vi "MecanumRobot.vi"() -> ()   [LabVIEW 2019]
uses:
  <vilib>/MakerHub/Xbox-One-Controller/Public/Open First Controller.vi
  <vilib>/vision/driver/NI_Vision_Acquisition_Software.lvlib
  <vilib>/MakerHub/Xbox-One-Controller/Private/Type Defs/Indicators/DPad Enum.ctl
  <vilib>/MakerHub/Xbox-One-Controller/Private/Type Defs/Indicators/All Axis Data.ctl
panel:
  out "SALIDA 4":string
  in  "Tab Control":enum32{"JOYSTICK", "COMUNICACION", "CAMARA"}(tab)
  out "A":bool
  out "AB":bool
  out "B":bool
  out "stay":bool
  out "Reverse":bool
  out "Forward":bool
  out "Left":bool
  out "Right":bool
  out "RL":bool
  out "FR":bool
  out "RR":bool
  out "FL":bool
  out "All Axis":T1
  out "Boolean":bool
  in  "Boton Prueba":bool
  in  "BOTON A":bool
  out "SALIDA":string
  out "SALIDA 2":string
  in  "address":string="192.168.0.16"
  out "SALIDA 3":string
  in  "stop":bool
  in  "DETENER EL PROGRAMA":bool
  out "Buffer Number":u32
  out "Frame Rate":dbl(knob) scale=0.0..100.0
  in  "Stop":bool
  in  "Camera Name":refnum<k21> caption="IMAQdx Session"
  out "Image":T3(plugin-control)
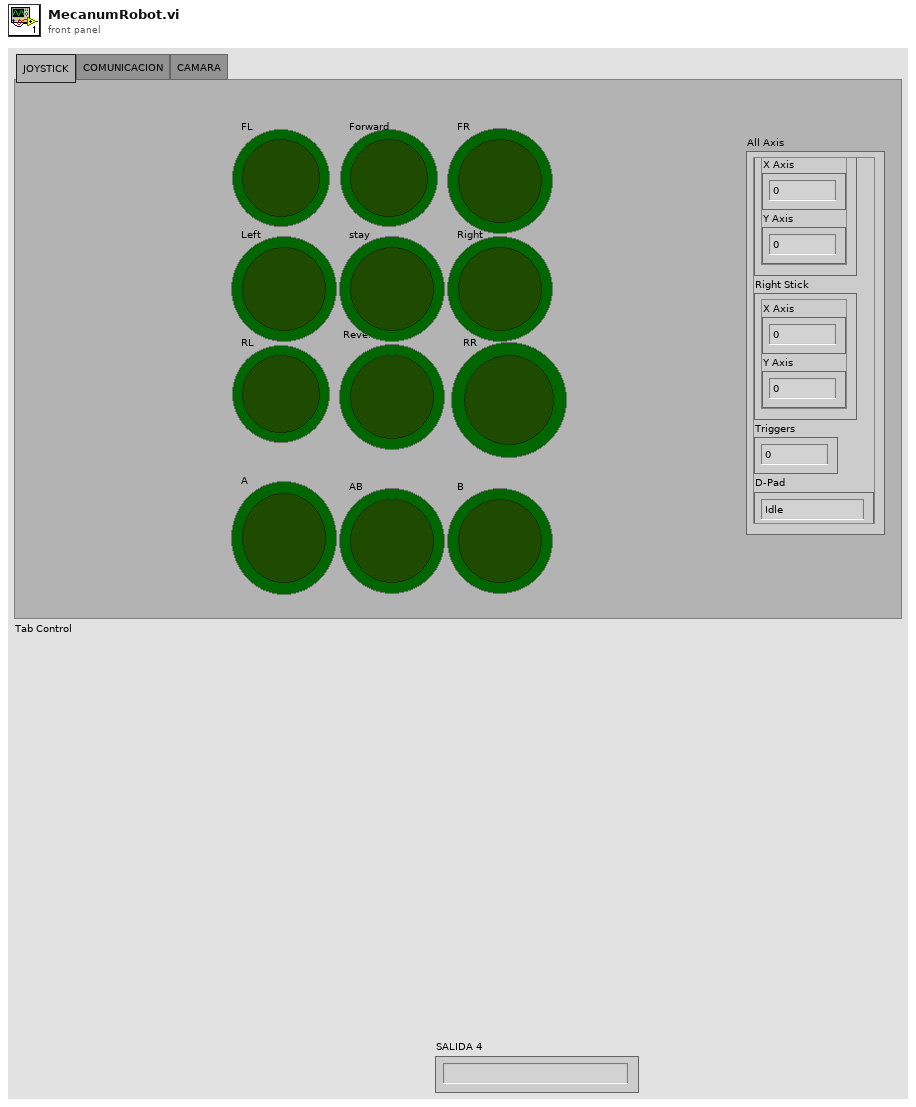
[diagram p1: front panel]
types:
  T1 = typedef "LMH-Xbox-One-Controller.lvlib/All Axis Data.ctl" = cluster{"Left Stick":cluster{"X Axis":i32, "Y Axis":i32}, "Right Stick":cluster{"X Axis":i32, "Y Axis":i32}, "Triggers":i32, "D-Pad":T2}
  T2 = typedef "LMH-Xbox-One-Controller.lvlib/DPad Enum.ctl" = enum16{"Idle", "Up", "Up / Right", "Right", "Down / Right", "Down", "Down / Left", "Left", "Up / Left"}
  T3 = typedef "IMAQ Image.ctl" = refnum<image>
  T4 = typedef "LMH-Xbox-One-Controller.lvlib/Xbox One Controller Ref.ctl" = cluster{"Controller Ref":refnum<k1>, "Event Refnum":refnum<event-registration>, "Worker Ref":refnum<vi>}
  T5 = typedef "IMAQdx.ctl" = refnum<k21>
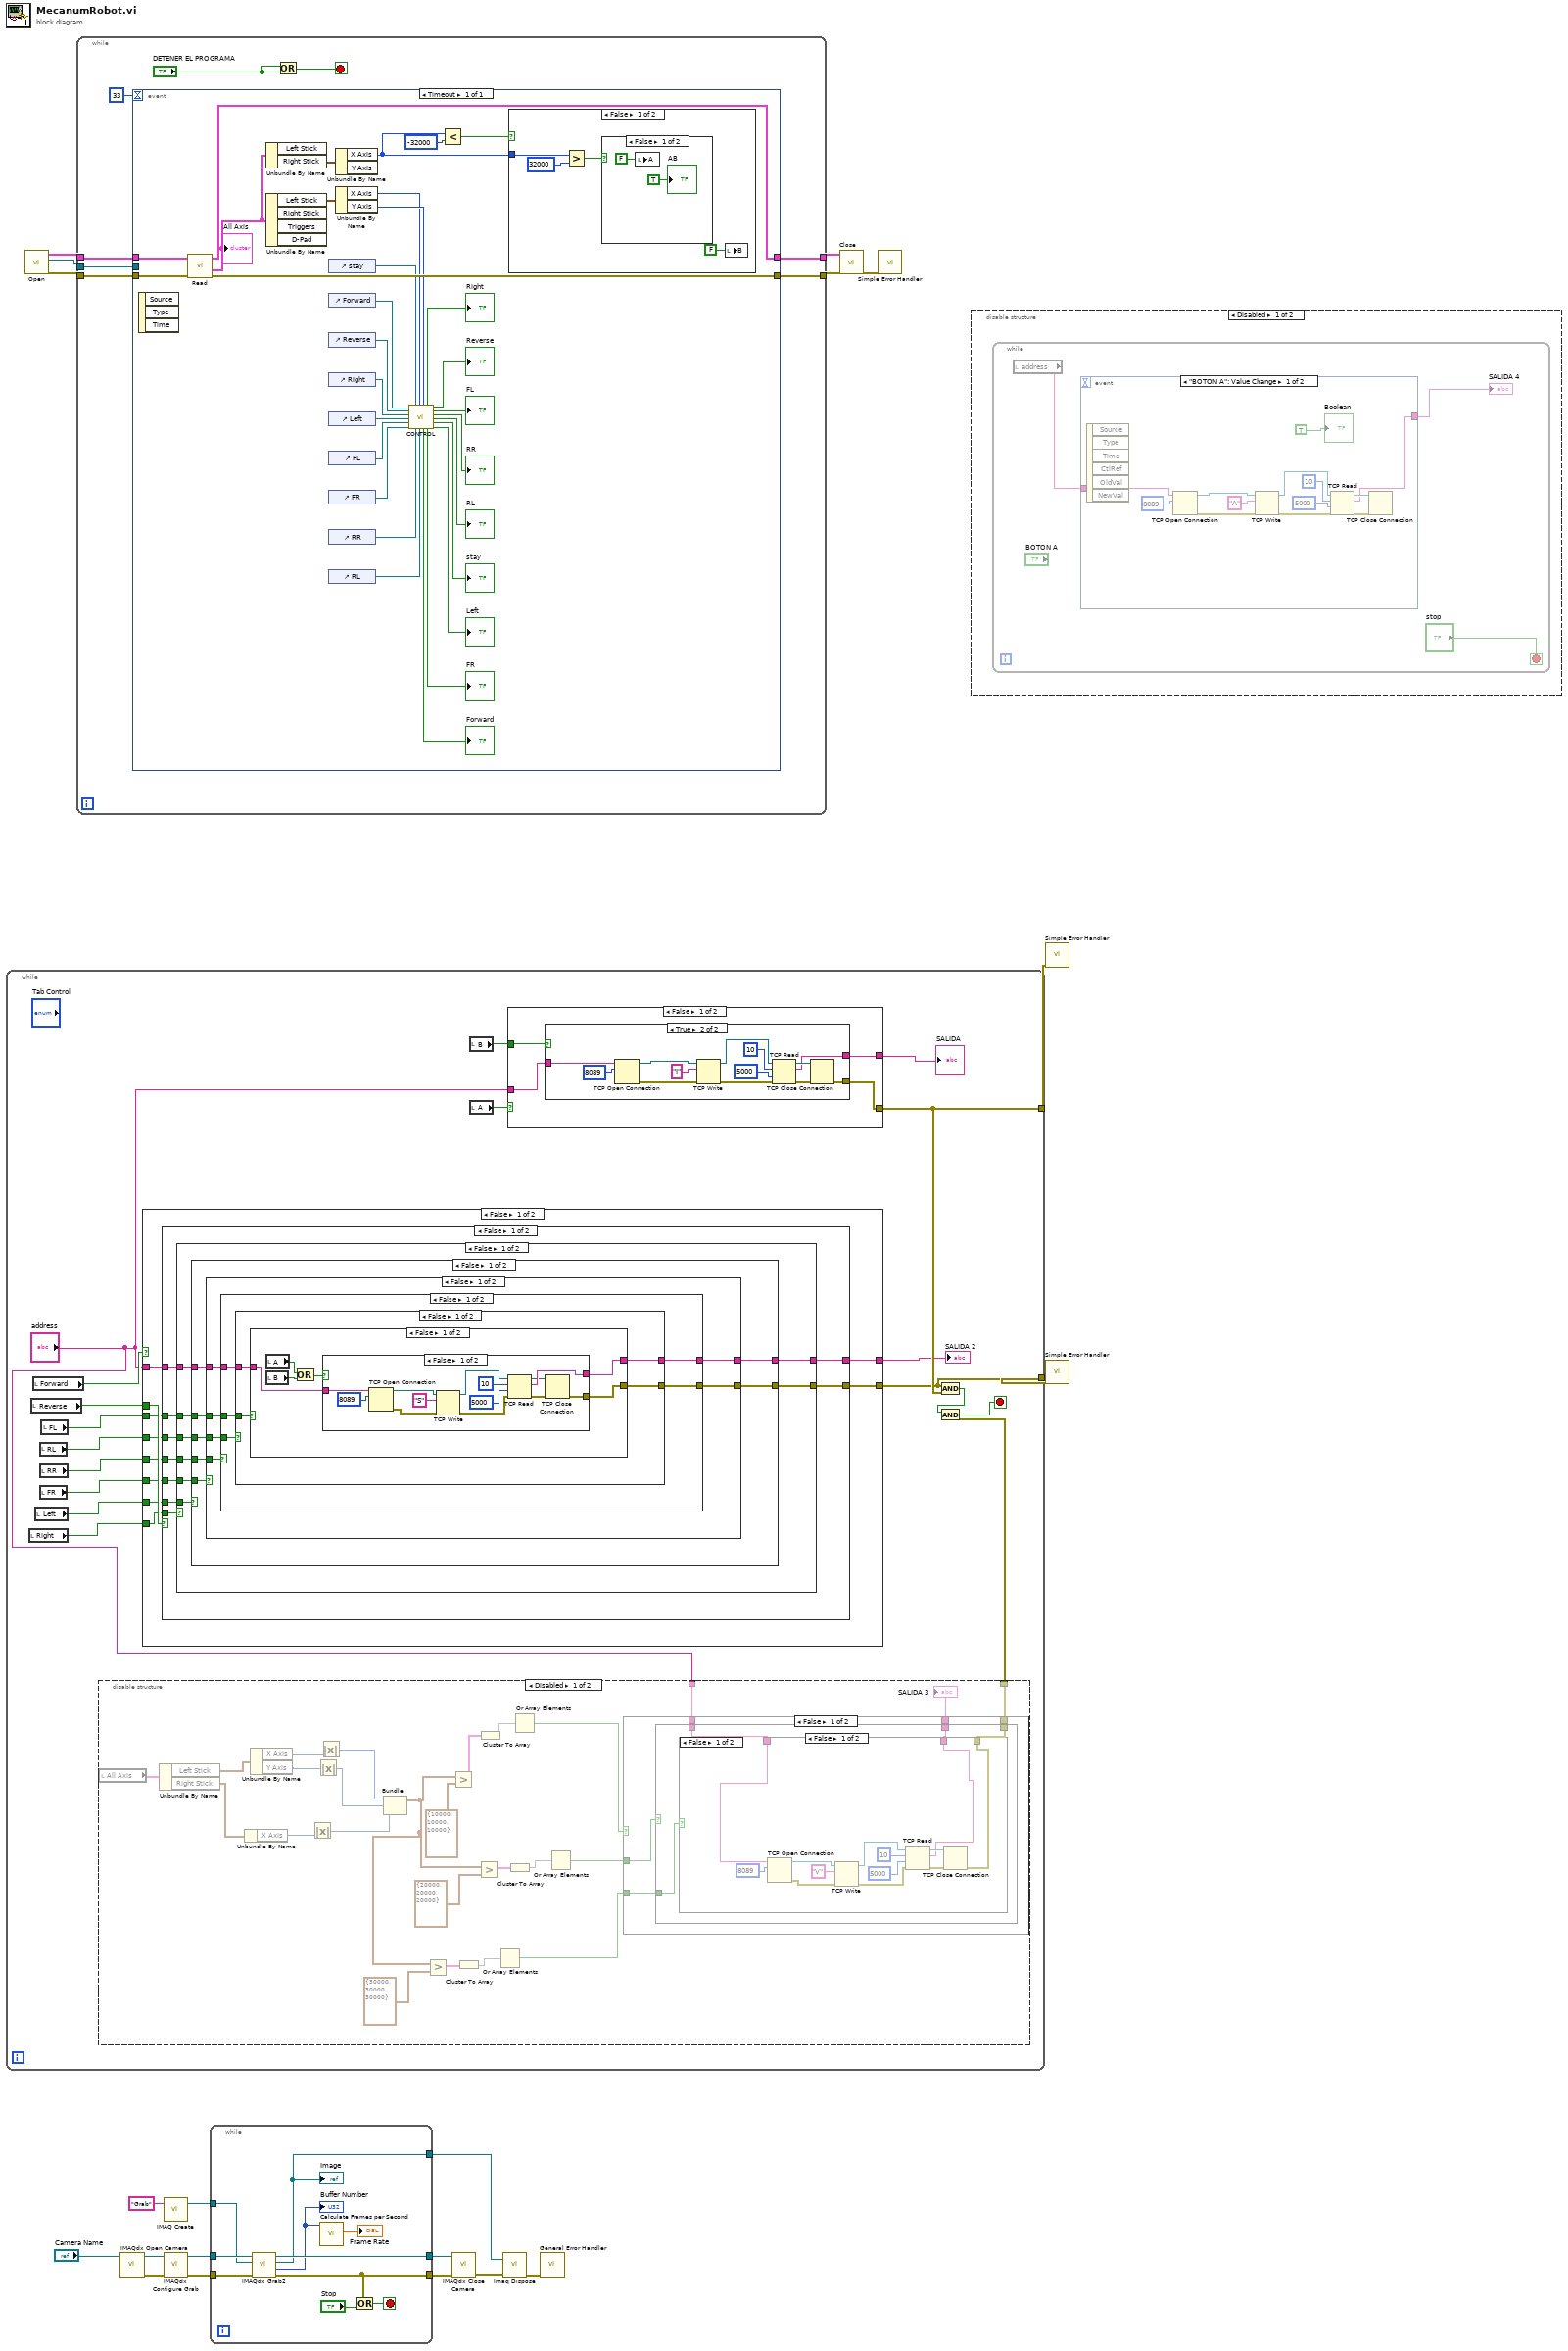
[diagram p0: block diagram]
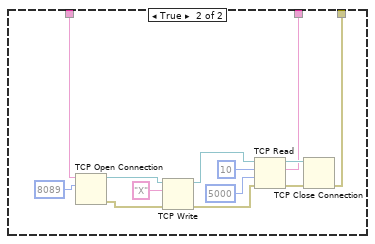
[diagram p2: hidden frame]
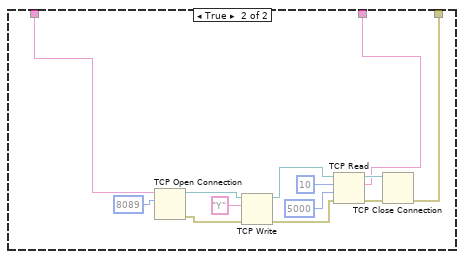
[diagram p3: hidden frame]
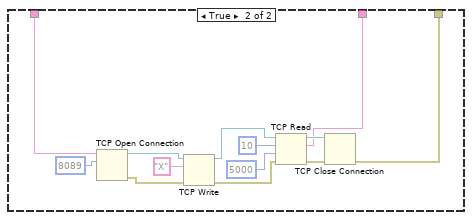
[diagram p4: hidden frame]
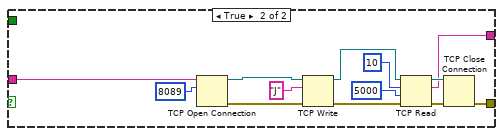
[diagram p7: hidden frame]
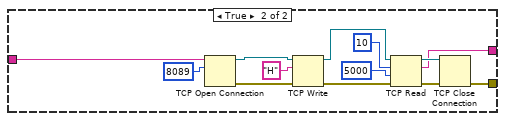
[diagram p9: hidden frame]
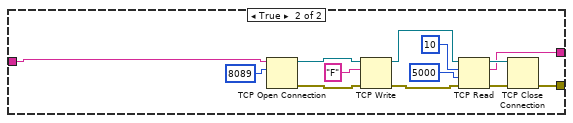
[diagram p10: hidden frame]
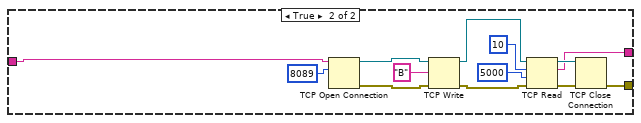
[diagram p11: hidden frame]
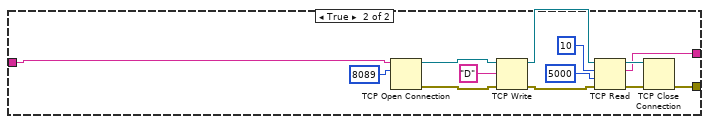
[diagram p12: hidden frame]
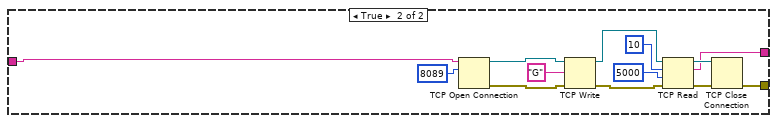
[diagram p13: hidden frame]
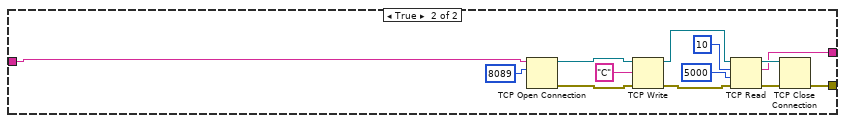
[diagram p14: hidden frame]
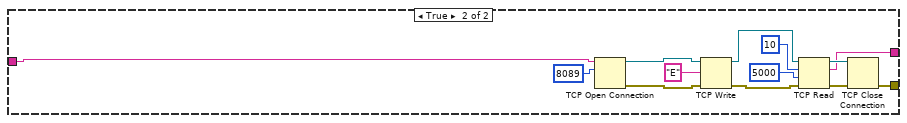
[diagram p15: hidden frame]
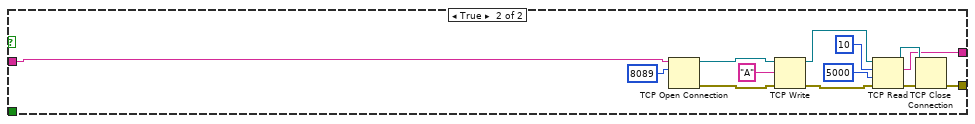
[diagram p16: hidden frame]
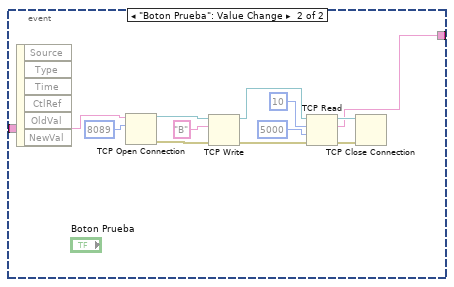
[diagram p17: hidden frame]
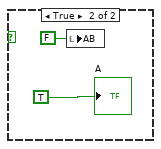
[diagram p19: hidden frame]
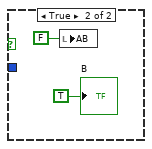
[diagram p20: hidden frame]
diagram:
  n1 = while {
    tunnel: [w28] -> w13
    tunnel: [w29] -> w14
    stop <- w21 stop-if-true
    n2 = local read "Right"() -> (w36:bool)
    n3 = local read "Reverse"() -> (w37:bool)
    n4 = local read "Forward"() -> (w38:bool)
    n5 = local read "Left"() -> (w35:bool)
    n6 = local read "RL"() -> (w32:bool)
    n7 = local read "RR"() -> (w33:bool)
    n8 = local read "FR"() -> (w34:bool)
    n9 = local read "FL"() -> (w31:bool)
    n10 = disable-structure shown="Disabled" {
      disable-tunnel: "address" -> [w63 _]
      disable-tunnel: [w62 _] -> w22
      frame Disabled {
        n11 = local read "All Axis"() -> (w61:T1)
        n12 = Unbundle By Name(w61) -> ("Left Stick"=w60:cluster{"X Axis":i32, "Y Axis":i32}, "Right Stick"=w59:cluster{"X Axis":i32, "Y Axis":i32})
        n13 = Unbundle By Name(w59) -> ("X Axis"=w53:i32)
        n14 = Unbundle By Name(w60) -> ("X Axis"=w58:i32, "Y Axis"=w57:i32)
        n15 = Absolute Value(x=w53) -> (abs(x)=w54:i32)
        n16 = Absolute Value(x=w57) -> (abs(x)=w55:i32)
        n17 = Absolute Value(x=w58) -> (abs(x)=w56:i32)
        n18 = Bundle(w56, w55, w54) -> (w43:cluster{i32, i32, i32})  [unwired: 1 in]
        n19 = Greater?(x=w43, y=cluster{i32, i32, i32} {30000, 30000, 30000}) -> (0:w45:cluster{bool, bool, bool})
        n20 = Greater?(x=w43, y=cluster{i32, i32, i32} {10000, 10000, 10000}) -> (0:w51:cluster{bool, bool, bool})
        n21 = Cluster To Array(cluster=w45) -> (array=w44:bool[])
        n22 = Greater?(x=w43, y=cluster{i32, i32, i32} {20000, 20000, 20000}) -> (0:w48:cluster{bool, bool, bool})
        n23 = Cluster To Array(cluster=w51) -> (array=w50:bool[])
        n24 = Or Array Elements(Boolean array=w44) -> (logical OR=w39:bool)
        n25 = Cluster To Array(cluster=w48) -> (array=w47:bool[])
        n26 = Or Array Elements(Boolean array=w50) -> (logical OR=w42:bool)
        n27 = Or Array Elements(Boolean array=w47) -> (logical OR=w40:bool)
        n28 = case shown="False" w42 {
          tunnel: w63 -> [w66 w114]
          tunnel: [w68 w113] -> w62
          tunnel: [w67 w112] -> w41
          tunnel: w40 -> [w65 _]
          tunnel: w39 -> [w64 _]
          frame False {
            n29 = case shown="False" w65 {
              tunnel: [w70 w101] -> w68
              tunnel: [w71 w100] -> w67
              tunnel: w66 -> [w69 w99]
              tunnel: w64 -> [w72 _]
              frame False {
                n30 = case shown="False" w72 {
                  tunnel: [w74 w88] -> w71
                  tunnel: [w75 w87] -> w70
                  tunnel: w69 -> [w73 w86]
                  frame False {
                    n31 = TCP Open Connection(address=w73, remote port or service name=u16 8089) -> (connection ID=w80:refnum<k5>, error out=w79:errorcluster)  [unwired: 3 in]
                    n32 = TCP Write(connection ID=w80, data in="V", error in (no error)=w79) -> (connection ID out=w83:refnum<k5>, error out=w82:errorcluster)  [unwired: 1 in, 1 out]
                    n33 = TCP Read(connection ID=w83, bytes to read=10, error in (no error)=w82, 9:5000 ("timeout ms (25000)")) -> (connection ID out=w78:refnum<k5>, data out=w74:string, error out=w77:errorcluster)  [unwired: 1 in]
                    n34 = TCP Close Connection(connection ID=w78, error in (no error)=w77) -> (error out=w75:errorcluster)  [unwired: 1 in, 1 out]
                  }
                  frame True {
                    n35 = TCP Open Connection(address=w86, remote port or service name=u16 8089) -> (connection ID=w95:refnum<k5>, error out=w96:errorcluster)  [unwired: 3 in]
                    n36 = TCP Write(connection ID=w95, data in="X", error in (no error)=w96) -> (connection ID out=w93:refnum<k5>, error out=w94:errorcluster)  [unwired: 1 in, 1 out]
                    n37 = TCP Read(connection ID=w93, bytes to read=10, error in (no error)=w94, 9:5000 ("timeout ms (25000)")) -> (connection ID out=w97:refnum<k5>, data out=w88:string, error out=w98:errorcluster)  [unwired: 1 in]
                    n38 = TCP Close Connection(connection ID=w97, error in (no error)=w98) -> (error out=w87:errorcluster)  [unwired: 1 in, 1 out]
                  }
                }
              }
              frame True {
                n39 = TCP Open Connection(address=w99, remote port or service name=u16 8089) -> (connection ID=w106:refnum<k5>, error out=w105:errorcluster)  [unwired: 3 in]
                n40 = TCP Write(connection ID=w106, data in="Y", error in (no error)=w105) -> (connection ID out=w109:refnum<k5>, error out=w108:errorcluster)  [unwired: 1 in, 1 out]
                n41 = TCP Read(connection ID=w109, bytes to read=10, error in (no error)=w108, 9:5000 ("timeout ms (25000)")) -> (connection ID out=w104:refnum<k5>, data out=w100:string, error out=w103:errorcluster)  [unwired: 1 in]
                n42 = TCP Close Connection(connection ID=w104, error in (no error)=w103) -> (error out=w101:errorcluster)  [unwired: 1 in, 1 out]
              }
            }
          }
          frame True {
            n43 = TCP Open Connection(address=w114, remote port or service name=u16 8089) -> (connection ID=w119:refnum<k5>, error out=w118:errorcluster)  [unwired: 3 in]
            n44 = TCP Write(connection ID=w119, data in="X", error in (no error)=w118) -> (connection ID out=w122:refnum<k5>, error out=w121:errorcluster)  [unwired: 1 in, 1 out]
            n45 = TCP Read(connection ID=w122, bytes to read=10, error in (no error)=w121, 9:5000 ("timeout ms (25000)")) -> (connection ID out=w117:refnum<k5>, data out=w112:string, error out=w116:errorcluster)  [unwired: 1 in]
            n46 = TCP Close Connection(connection ID=w117, error in (no error)=w116) -> (error out=w113:errorcluster)  [unwired: 1 in, 1 out]
          }
        }
        "SALIDA 3" <- w41
      }
      frame Enabled {
      }
    }
    n47 = case shown="False" w38 {
      tunnel: [w164 w316] -> w28
      tunnel: w37 -> [w163 _]
      tunnel: "address" -> [w162 w315]
      tunnel: w36 -> [w161 _]
      tunnel: w35 -> [w160 _]
      tunnel: w34 -> [w159 _]
      tunnel: w33 -> [w158 _]
      tunnel: w32 -> [w157 _]
      tunnel: w31 -> [w156 _]
      tunnel: [w155 w314] -> w26
      frame False {
        n48 = case shown="False" w163 {
          tunnel: [w172 w303] -> w164
          tunnel: w162 -> [w173 w302]
          tunnel: w161 -> [w171 _]
          tunnel: w160 -> [w170 _]
          tunnel: w159 -> [w169 _]
          tunnel: w158 -> [w168 _]
          tunnel: w157 -> [w167 _]
          tunnel: w156 -> [w166 _]
          tunnel: [w165 w301] -> w155
          frame False {
            n49 = case shown="False" w171 {
              tunnel: w173 -> [w181 w290]
              tunnel: [w180 w289] -> w172
              tunnel: w170 -> [w179 _]
              tunnel: w169 -> [w178 _]
              tunnel: w168 -> [w177 _]
              tunnel: w167 -> [w176 _]
              tunnel: w166 -> [w175 _]
              tunnel: [w174 w288] -> w165
              frame False {
                n50 = case shown="False" w179 {
                  tunnel: w181 -> [w188 w278]
                  tunnel: [w186 w276] -> w180
                  tunnel: w178 -> [w187 _]
                  tunnel: w177 -> [w185 _]
                  tunnel: w176 -> [w184 _]
                  tunnel: w175 -> [w183 _]
                  tunnel: [w182 w275] -> w174
                  frame False {
                    n51 = case shown="False" w187 {
                      tunnel: w188 -> [w193 w264]
                      tunnel: [w194 w263] -> w186
                      tunnel: w185 -> [w192 _]
                      tunnel: w184 -> [w191 _]
                      tunnel: w183 -> [w190 _]
                      tunnel: [w189 w262] -> w182
                      frame False {
                        n52 = case shown="False" w192 {
                          tunnel: [w199 w251] -> w194
                          tunnel: w193 -> [w198 w250]
                          tunnel: w191 -> [w197 _]
                          tunnel: w190 -> [w196 _]
                          tunnel: [w195 w249] -> w189
                          frame False {
                            n53 = case shown="False" w197 {
                              tunnel: [w203 w238] -> w199
                              tunnel: w198 -> [w201 w237]
                              tunnel: w196 -> [w202 _]
                              tunnel: [w200 w236] -> w195
                              frame False {
                                n54 = case shown="False" w202 {
                                tunnel: [w208 w225] -> w203
                                tunnel: w201 -> [w209 w224]
                                tunnel: [w207 w223] -> w200
                                frame False {
                                n55 = local read "A"() -> (w205:bool)
                                n56 = local read "B"() -> (w204:bool)
                                n57 = Or(x=w205, y=w204) -> (x .or. y?=w206:bool)
                                n58 = case shown="False" w206 {
                                tunnel: w209 -> [w222 _]
                                tunnel: [w221 _] -> w208
                                tunnel: [w220 _] -> w207
                                frame False {
                                n59 = TCP Open Connection(address=w222, remote port or service name=u16 8089) -> (connection ID=w214:refnum<k5>, error out=w213:errorcluster)  [unwired: 3 in]
                                n60 = TCP Write(connection ID=w214, data in="S", error in (no error)=w213) -> (connection ID out=w217:refnum<k5>, error out=w216:errorcluster)  [unwired: 1 in, 1 out]
                                n61 = TCP Read(connection ID=w217, bytes to read=10, error in (no error)=w216, 9:5000 ("timeout ms (25000)")) -> (connection ID out=w212:refnum<k5>, data out=w220:string, error out=w211:errorcluster)  [unwired: 1 in]
                                n62 = TCP Close Connection(connection ID=w212, error in (no error)=w211) -> (error out=w221:errorcluster)  [unwired: 1 in, 1 out]
                                }
                                frame True {
                                }
                                }
                                }
                                frame True {
                                n63 = TCP Open Connection(address=w224, remote port or service name=u16 8089) -> (connection ID=w230:refnum<k5>, error out=w229:errorcluster)  [unwired: 3 in]
                                n64 = TCP Write(connection ID=w230, data in="H", error in (no error)=w229) -> (connection ID out=w233:refnum<k5>, error out=w232:errorcluster)  [unwired: 1 in, 1 out]
                                n65 = TCP Read(connection ID=w233, bytes to read=10, error in (no error)=w232, 9:5000 ("timeout ms (25000)")) -> (connection ID out=w228:refnum<k5>, data out=w223:string, error out=w227:errorcluster)  [unwired: 1 in]
                                n66 = TCP Close Connection(connection ID=w228, error in (no error)=w227) -> (error out=w225:errorcluster)  [unwired: 1 in, 1 out]
                                }
                                }
                              }
                              frame True {
                                n67 = TCP Open Connection(address=w237, remote port or service name=u16 8089) -> (connection ID=w243:refnum<k5>, error out=w242:errorcluster)  [unwired: 3 in]
                                n68 = TCP Write(connection ID=w243, data in="F", error in (no error)=w242) -> (connection ID out=w246:refnum<k5>, error out=w245:errorcluster)  [unwired: 1 in, 1 out]
                                n69 = TCP Read(connection ID=w246, bytes to read=10, error in (no error)=w245, 9:5000 ("timeout ms (25000)")) -> (connection ID out=w241:refnum<k5>, data out=w236:string, error out=w240:errorcluster)  [unwired: 1 in]
                                n70 = TCP Close Connection(connection ID=w241, error in (no error)=w240) -> (error out=w238:errorcluster)  [unwired: 1 in, 1 out]
                              }
                            }
                          }
                          frame True {
                            n71 = TCP Open Connection(address=w250, remote port or service name=u16 8089) -> (connection ID=w258:refnum<k5>, error out=w259:errorcluster)  [unwired: 3 in]
                            n72 = TCP Write(connection ID=w258, data in="B", error in (no error)=w259) -> (connection ID out=w256:refnum<k5>, error out=w257:errorcluster)  [unwired: 1 in, 1 out]
                            n73 = TCP Read(connection ID=w256, bytes to read=10, error in (no error)=w257, 9:5000 ("timeout ms (25000)")) -> (connection ID out=w260:refnum<k5>, data out=w249:string, error out=w261:errorcluster)  [unwired: 1 in]
                            n74 = TCP Close Connection(connection ID=w260, error in (no error)=w261) -> (error out=w251:errorcluster)  [unwired: 1 in, 1 out]
                          }
                        }
                      }
                      frame True {
                        n75 = TCP Open Connection(address=w264, remote port or service name=u16 8089) -> (connection ID=w271:refnum<k5>, error out=w272:errorcluster)  [unwired: 3 in]
                        n76 = TCP Write(connection ID=w271, data in="D", error in (no error)=w272) -> (connection ID out=w269:refnum<k5>, error out=w270:errorcluster)  [unwired: 1 in, 1 out]
                        n77 = TCP Read(connection ID=w269, bytes to read=10, error in (no error)=w270, 9:5000 ("timeout ms (25000)")) -> (connection ID out=w273:refnum<k5>, data out=w262:string, error out=w274:errorcluster)  [unwired: 1 in]
                        n78 = TCP Close Connection(connection ID=w273, error in (no error)=w274) -> (error out=w263:errorcluster)  [unwired: 1 in, 1 out]
                      }
                    }
                  }
                  frame True {
                    n79 = TCP Open Connection(address=w278, remote port or service name=u16 8089) -> (connection ID=w282:refnum<k5>, error out=w281:errorcluster)  [unwired: 3 in]
                    n80 = TCP Write(connection ID=w282, data in="G", error in (no error)=w281) -> (connection ID out=w285:refnum<k5>, error out=w284:errorcluster)  [unwired: 1 in, 1 out]
                    n81 = TCP Read(connection ID=w285, bytes to read=10, error in (no error)=w284, 9:5000 ("timeout ms (25000)")) -> (connection ID out=w280:refnum<k5>, data out=w275:string, error out=w279:errorcluster)  [unwired: 1 in]
                    n82 = TCP Close Connection(connection ID=w280, error in (no error)=w279) -> (error out=w276:errorcluster)  [unwired: 1 in, 1 out]
                  }
                }
              }
              frame True {
                n83 = TCP Open Connection(address=w290, remote port or service name=u16 8089) -> (connection ID=w294:refnum<k5>, error out=w293:errorcluster)  [unwired: 3 in]
                n84 = TCP Write(connection ID=w294, data in="C", error in (no error)=w293) -> (connection ID out=w298:refnum<k5>, error out=w297:errorcluster)  [unwired: 1 in, 1 out]
                n85 = TCP Read(connection ID=w298, bytes to read=10, error in (no error)=w297, 9:5000 ("timeout ms (25000)")) -> (connection ID out=w292:refnum<k5>, data out=w288:string, error out=w291:errorcluster)  [unwired: 1 in]
                n86 = TCP Close Connection(connection ID=w292, error in (no error)=w291) -> (error out=w289:errorcluster)  [unwired: 1 in, 1 out]
              }
            }
          }
          frame True {
            n87 = TCP Open Connection(address=w302, remote port or service name=u16 8089) -> (connection ID=w307:refnum<k5>, error out=w306:errorcluster)  [unwired: 3 in]
            n88 = TCP Write(connection ID=w307, data in="E", error in (no error)=w306) -> (connection ID out=w311:refnum<k5>, error out=w310:errorcluster)  [unwired: 1 in, 1 out]
            n89 = TCP Read(connection ID=w311, bytes to read=10, error in (no error)=w310, 9:5000 ("timeout ms (25000)")) -> (connection ID out=w305:refnum<k5>, data out=w301:string, error out=w304:errorcluster)  [unwired: 1 in]
            n90 = TCP Close Connection(connection ID=w305, error in (no error)=w304) -> (error out=w303:errorcluster)  [unwired: 1 in, 1 out]
          }
        }
      }
      frame True {
        n91 = TCP Open Connection(address=w315, remote port or service name=u16 8089) -> (connection ID=w320:refnum<k5>, error out=w319:errorcluster)  [unwired: 3 in]
        n92 = TCP Write(connection ID=w320, data in="A", error in (no error)=w319) -> (connection ID out=w324:refnum<k5>, error out=w323:errorcluster)  [unwired: 1 in, 1 out]
        n93 = TCP Read(connection ID=w324, bytes to read=10, error in (no error)=w323, 9:5000 ("timeout ms (25000)")) -> (connection ID out=w318:refnum<k5>, data out=w314:string, error out=w317:errorcluster)  [unwired: 1 in]
        n94 = TCP Close Connection(connection ID=w318, error in (no error)=w317) -> (error out=w316:errorcluster)  [unwired: 1 in, 1 out]
      }
    }
    "SALIDA 2" <- w26
    n95 = local read "B"() -> (w27:bool)
    n96 = local read "A"() -> (w30:bool)
    n97 = case shown="False" w30 {
      tunnel: [w126 w144] -> w29
      tunnel: "address" -> [w127 w143]
      tunnel: w27 -> [w128 _]
      tunnel: [w125 w142] -> w25
      frame False {
        n98 = case shown="True" w128 {
          tunnel: w127 -> [_ w131]
          tunnel: [_ w130] -> w126
          tunnel: [_ w129] -> w125
          frame False {
          }
          frame True {
            n99 = TCP Open Connection(address=w131, remote port or service name=u16 8089) -> (connection ID=w139:refnum<k5>, error out=w138:errorcluster)  [unwired: 3 in]
            n100 = TCP Write(connection ID=w139, data in="I", error in (no error)=w138) -> (connection ID out=w141:refnum<k5>, error out=w140:errorcluster)  [unwired: 1 in, 1 out]
            n101 = TCP Read(connection ID=w141, bytes to read=10, error in (no error)=w140, 9:5000 ("timeout ms (25000)")) -> (connection ID out=w137:refnum<k5>, data out=w129:string, error out=w136:errorcluster)  [unwired: 1 in]
            n102 = TCP Close Connection(connection ID=w137, error in (no error)=w136) -> (error out=w130:errorcluster)  [unwired: 1 in, 1 out]
          }
        }
      }
      frame True {
        n103 = TCP Open Connection(address=w143, remote port or service name=u16 8089) -> (connection ID=w151:refnum<k5>, error out=w152:errorcluster)  [unwired: 3 in]
        n104 = TCP Write(connection ID=w151, data in="J", error in (no error)=w152) -> (connection ID out=w149:refnum<k5>, error out=w150:errorcluster)  [unwired: 1 in, 1 out]
        n105 = TCP Read(connection ID=w149, bytes to read=10, error in (no error)=w150, 9:5000 ("timeout ms (25000)")) -> (connection ID out=w153:refnum<k5>, data out=w142:string, error out=w154:errorcluster)  [unwired: 1 in]
        n106 = TCP Close Connection(connection ID=w153, error in (no error)=w154) -> (error out=w144:errorcluster)  [unwired: 1 in, 1 out]
      }
    }
    "SALIDA" <- w25
    n107 = And(x=w28, y=w29) -> (x .and. y?=w23:bool)
    n108 = And(x=w23, y=w22) -> (x .and. y?=w21:bool)
  }
  n109 = call-poly <vilib>:"Open.vi"() -> ("Error Out"=w18:errorcluster, "Event Refnum"=w19:refnum<event-registration>, "Xbox One Controller"=w20:T4)  [unwired: 9 in]
  n110 = while {
    tunnel: w20 -> [w334]
    tunnel: w19 -> [w333]
    tunnel: w18 -> [w332]
    tunnel: [w331] -> w17
    tunnel: [w330] -> w16
    stop <- w328 stop-if-true
    n111 = event shown="[0] Timeout" {
      selector: _ -> [_]
      dyn-events: _ -> [_]
      timeout: 33 -> [_]
      tunnel: w334 -> [w363]
      tunnel: w333 -> [_]
      tunnel: w332 -> [w364]
      tunnel: [w340] -> w331
      tunnel: [w362] -> w330
      event Timeout {
        n112 = event-data() -> ()  [unwired: 1 in, 3 out]
        n113 = call <vilib>:"Read.vi"("Error In"=w364, "Xbox One Controller Ref"=w363) -> ("Error Out"=w362:errorcluster, "All Axis"=w339:T1, "Xbox One Controller Ref"=w340:T4)  [unwired: 6 in, 1 out]
        "All Axis" <- w339
        n114 = Unbundle By Name(w339) -> ("Right Stick"=w338:cluster{"X Axis":i32, "Y Axis":i32})  [unwired: 1 out]
        n115 = Unbundle By Name(w339) -> ("Left Stick"=w361:cluster{"X Axis":i32, "Y Axis":i32})  [unwired: 3 out]
        n116 = control-ref of="stay"() -> (w351:refnum<vi>)
        n117 = control-ref of="Forward"() -> (w350:refnum<vi>)
        n118 = control-ref of="Reverse"() -> (w358:refnum<vi>)
        n119 = control-ref of="Right"() -> (w357:refnum<vi>)
        n120 = control-ref of="Left"() -> (w356:refnum<vi>)
        n121 = control-ref of="FL"() -> (w355:refnum<vi>)
        n122 = control-ref of="FR"() -> (w354:refnum<vi>)
        n123 = control-ref of="RR"() -> (w353:refnum<vi>)
        n124 = control-ref of="RL"() -> (w352:refnum<vi>)
        n125 = Unbundle By Name(w338) -> ("X Axis"=w335:i32)  [unwired: 1 out]
        n126 = Unbundle By Name(w361) -> ("X Axis"=w359:i32, "Y Axis"=w360:i32)
        n127 = call "CONTROL.vi"("Boolean in"=w350, "reference"=w358, "reference 2"=w357, "reference 3"=w356, "reference 4"=w355, "reference 5"=w354, "reference 8"=w351, "reference 6"=w353, "X Axis"=w359, "reference 7"=w352, "Y Axis"=w360) -> ("Foward"=→"Forward":bool, "Right"=→"Right":bool, "FR"=→"FR":bool, "Reverse"=→"Reverse":bool, "FL"=→"FL":bool, "RR"=→"RR":bool, "RL"=→"RL":bool, "stay"=→"stay":bool, "Left"=→"Left":bool)
        n128 = Less?(x=w335, y=-32000) -> (x < y?=w336:bool)
        n129 = case shown="False" w336 {
          tunnel: w335 -> [w368 _]
          frame False {
            n130 = Greater?(x=w368, y=32000) -> (0:w366:bool)
            n131 = case shown="False" w366 {
              frame False {
                n132 = local write "A"(FALSE ("A")) -> ()
                "AB" <- TRUE ("AB")
              }
              frame True {
                n133 = local write "AB"(FALSE ("AB")) -> ()
                "A" <- TRUE ("A")
              }
            }
            n134 = local write "B"(FALSE ("A")) -> ()
          }
          frame True {
            n135 = local write "AB"(FALSE ("AB")) -> ()
            "B" <- TRUE ("B")
          }
        }
      }
    }
    n136 = Or(x="DETENER EL PROGRAMA", y="DETENER EL PROGRAMA") -> (x .or. y?=w328:bool)
  }
  n137 = call <vilib>:"IMAQdx Open Camera.vi"("Session In"="Camera Name") -> ("error out"=w7:errorcluster, "Session Out"=w6:T5)  [unwired: 2 in, 7 out]
  n138 = call "IMAQ Create"("Image Name"="Grab") -> ("New Image"=w12:T3)  [unwired: 3 in, 2 out]
  n139 = call <vilib>:"IMAQdx Configure Grab.vi"("error in"=w7, "Session In"=w6) -> ("error out"=w10:errorcluster, "Session Out"=w11:T5)  [unwired: 1 in, 7 out]
  n140 = while {
    tunnel: [w379] -> w9
    tunnel: w10 -> [w381]
    tunnel: w11 -> [w382]
    tunnel: [w376] -> w8
    tunnel: w12 -> [w380]
    tunnel: [w375] -> w4
    stop <- w384 stop-if-true
    n141 = call <vilib>:"IMAQdx Grab2.vi"("error in"=w381, "Image In"=w380, "Session In"=w382) -> ("error out"=w376:errorcluster, "Buffer Number Out"=w377:u32, "Image Out"=w375:T3, "Session Out"=w379:T5)  [unwired: 5 in]
    "Image" <- w375
    "Buffer Number" <- w377
    n142 = call <vilib>:"Calculate Frames per Second.vi"("Buffer Number"=w377) -> ("Processed Frames/s"=→"Frame Rate":dbl)  [unwired: 8 in, 2 out]
    n143 = Or(x=w376, y="Stop") -> (x .or. y?=w384:bool)
  }
  n144 = call <vilib>:"IMAQdx Close Camera.vi"("error in"=w8, "Session In"=w9) -> ("error out"=w3:errorcluster)  [unwired: 9 out]
  n145 = call "Imaq Dispose"("Image"=w4, "error in (no error)"=w3) -> ("error out"=w2:errorcluster)  [unwired: 4 in]
  n146 = call <vilib>:"General Error Handler.vi"("error in (no error)"=w2) -> ()  [unwired: 2 in, 13 out]
  n147 = call <vilib>:"Close.vi"("Error In"=w16, "Xbox One Controller Ref"=w17) -> ("Error Out"=w15:errorcluster)  [unwired: 9 in]
  n148 = call <vilib>:"Simple Error Handler.vi"("error in (no error)"=w15) -> ()  [unwired: 4 in, 5 out]
  n149 = disable-structure shown="Disabled" {
    frame Disabled {
      n150 = while {
        stop <- "stop" stop-if-true
        n151 = local read "address"() -> (w386:string)
        n152 = event shown="[0] \"BOTON A\": Value Change" {
          selector: _ -> [_ _]
          dyn-events: _ -> [_ _]
          timeout: _ -> [_ _]
          tunnel: [w390 w402] -> w387
          tunnel: w386 -> [w389 w401]
          event "BOTON A": Value Change {
            n153 = event-data() -> ()  [unwired: 1 in, 6 out]
            n154 = TCP Open Connection(address=w389, remote port or service name=u16 8089) -> (connection ID=w398:refnum<k5>, error out=w397:errorcluster)  [unwired: 3 in]
            n155 = TCP Write(connection ID=w398, data in="A", error in (no error)=w397) -> (connection ID out=w400:refnum<k5>, error out=w399:errorcluster)  [unwired: 1 in, 1 out]
            n156 = TCP Read(connection ID=w400, bytes to read=10, error in (no error)=w399, 9:5000 ("timeout ms (25000)")) -> (connection ID out=w396:refnum<k5>, data out=w390:string, error out=w395:errorcluster)  [unwired: 1 in]
            n157 = TCP Close Connection(connection ID=w396, error in (no error)=w395) -> ()  [unwired: 1 in, 2 out]
            "Boolean" <- TRUE ("Boolean")
          }
          event "Boton Prueba": Value Change {
            n158 = event-data() -> ()  [unwired: 1 in, 6 out]
            n159 = TCP Open Connection(address=w401, remote port or service name=u16 8089) -> (connection ID=w410:refnum<k5>, error out=w409:errorcluster)  [unwired: 3 in]
            n160 = TCP Write(connection ID=w410, data in="B", error in (no error)=w409) -> (connection ID out=w412:refnum<k5>, error out=w411:errorcluster)  [unwired: 1 in, 1 out]
            n161 = TCP Read(connection ID=w412, bytes to read=10, error in (no error)=w411, 9:5000 ("timeout ms (25000)")) -> (connection ID out=w408:refnum<k5>, data out=w402:string, error out=w407:errorcluster)  [unwired: 1 in]
            n162 = TCP Close Connection(connection ID=w408, error in (no error)=w407) -> ()  [unwired: 1 in, 2 out]
          }
        }
        "SALIDA 4" <- w387
      }
    }
    frame Enabled {
    }
  }
  n163 = call <vilib>:"Simple Error Handler.vi"("error in (no error)"=w14) -> ()  [unwired: 4 in, 5 out]
  n164 = call <vilib>:"Simple Error Handler.vi"("error in (no error)"=w13) -> ()  [unwired: 4 in, 5 out]
